vi "VI Tree.vi"() -> ()   [LabVIEW 2023, in "Label-Driven UI.lvlib"]
uses:
  Label-Driven UI.lvlib
  ef698b20-1dc8-4b30-883f-a444122f00d6.vi
  83c02c68-7d15-4879-bc89-eb71a368ed29.vi
  a679ed9e-7ae6-454f-bd91-6d61a8740d99.vi
  f0ebb126-57e9-4511-ad45-2aed94828c51.vi
  636c2352-9b1b-4e6b-a63f-5906ed7f56c4.vi
  da936bd9-5eef-46bc-870a-225bd0447414.vi
  7898772a-027b-481c-8fd9-68f4b24e3781.vi
panel:
  in  "error in":errorcluster
  in  "Nested in":refnum<class>
  # "VI Tree"
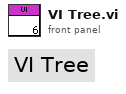
[diagram p1: front panel]
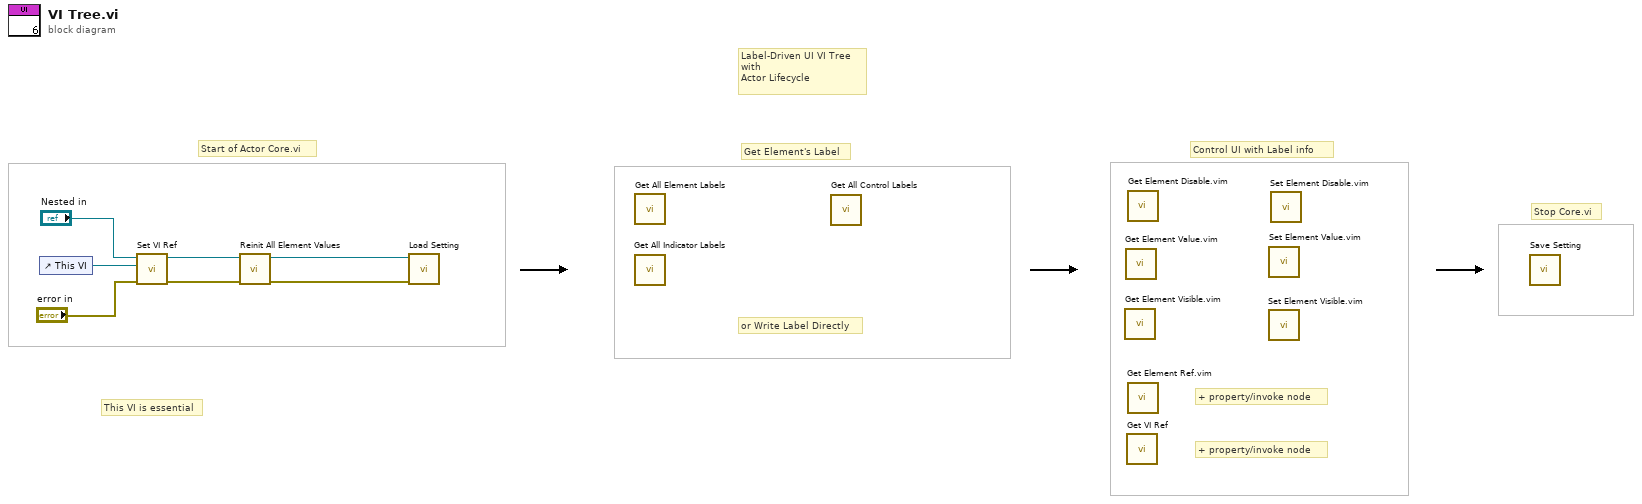
[diagram p0: block diagram]
diagram:
  # "or Write Label Directly"
  # "This VI is essential"
  # "Stop Core.vi"
  # "Get Element's Label"
  # "Control UI with Label info"
  # "+ property/invoke node"
  # "+ property/invoke node"
  # "Start of Actor Core.vi"
  # "Label-Driven UI VI Tree\nwith\nActor Lifecycle"
  n1 = control-ref of="This VI"() -> (w7:refnum<vi>)
  n2 = call "Set VI Ref.vi"("error in"="error in", "VI Refnum"=w7, "Class in"="Nested in") -> ("error out"=w4:errorcluster, "Class out"=w5:refnum<class>)  [unwired: 7 in]
  n3 = call "Reinit All Element Values.vi"("error in"=w4, "Class in"=w5) -> ("error out"=w2:errorcluster, "Class out"=w3:refnum<class>)  [unwired: 8 in]
  n4 = call "Load Setting.vi"("error in"=w2, "Class in"=w3) -> ()  [unwired: 8 in, 2 out]
  n5 = call "Get All Element Labels.vi"() -> ()  [unwired: 9 in, 3 out]
  n6 = call "Get All Indicator Labels.vi"() -> ()  [unwired: 9 in, 3 out]
  n7 = call "Get All Control Labels.vi"() -> ()  [unwired: 9 in, 3 out]
  n8 = call "Get Element Visible.vim"() -> ()  [unwired: 9 in, 3 out]
  n9 = call "Get Element Value.vim"() -> ()  [unwired: 9 in, 3 out]
  n10 = call "Get VI Ref.vi"() -> ()  [unwired: 9 in, 3 out]
  n11 = call "Get Element Disable.vim"() -> ()  [unwired: 9 in, 3 out]
  n12 = call "Get Element Ref.vim"() -> ()  [unwired: 9 in, 3 out]
  n13 = call "Set Element Value.vim"() -> ()  [unwired: 10 in, 2 out]
  n14 = call "Set Element Visible.vim"() -> ()  [unwired: 10 in, 2 out]
  n15 = call "Set Element Disable.vim"() -> ()  [unwired: 10 in, 2 out]
  n16 = call "Save Setting.vi"() -> ()  [unwired: 10 in, 2 out]
